vi "Read_WIP_All.vi"(7 "WIP In":i64[](array[numeric]), 8 "error in (no error)":errorcluster, 9 "WIP dIn":i64[](array[numeric]), 10 "Ref in":T1={"MS SQL Connection"=refnum, "UDL File"=path "", "Time"="", "DCODE"="", "WIP+1"=0, "MC No?"=0, "POKAYOKE?"=FALSE, "Expected Result"="", "Result [Status]"="", "Clock"=0.0, "RFID"="", "WIP Queue"=refnum, "TS Parameter"={"ProfitCenterCode"="", "LineCode"="", "WorkOrderNumber"="", "Model"="", "Model_with_Prefix"="", "VendorCode"="", "SetParameterDateCode"="", "PokaYoke"=0, "Target"=1, "Live_DateCode"="", "CustomerPartNumber"="", "Hand"="", "sBarcode"=FALSE, "FCA"=0, "Ent_Stamp"=timestamp(0 s since 1904-01-01), "STS_CD"=0.0}, "Data_Queue"=[], "RFID Serial No."=""} {"TS Parameter"."FCA" format="%01d"; "TS Parameter"."Target" min=1 max=100000; "TS Parameter"."PokaYoke" min=0 max=1}, 11 "Queue in":refnum<queue>) -> (0 "error out":errorcluster, 1 "WIP dOut":i64[](array[numeric]), 2 "Ref out":T1={"MS SQL Connection"=refnum, "UDL File"=path "", "Time"="", "DCODE"="", "WIP+1"=0, "MC No?"=0, "POKAYOKE?"=FALSE, "Expected Result"="", "Result [Status]"="", "Clock"=0.0, "RFID"="", "WIP Queue"=refnum, "TS Parameter"={"ProfitCenterCode"="", "LineCode"="", "WorkOrderNumber"="", "Model"="", "Model_with_Prefix"="", "VendorCode"="", "SetParameterDateCode"="", "PokaYoke"=0, "Target"=1, "Live_DateCode"="", "CustomerPartNumber"="", "Hand"="", "sBarcode"=FALSE, "FCA"=0, "Ent_Stamp"=timestamp(0 s since 1904-01-01), "STS_CD"=0.0}, "Data_Queue"=[], "RFID Serial No."=""} {"TS Parameter"."FCA" format="%01d"; "TS Parameter"."Target" min=1 max=100000; "TS Parameter"."PokaYoke" min=0 max=1}, 3 "Queue out":refnum<queue>, 4 "State Out":T4, 5 "WIP Out":i64[](array[numeric]))   [LabVIEW 2020]
uses:
  Controls/WIP_State.ctl
  Controls/TD SQL.ctl
  <vilib>/addons/database/Connection.llb/Conn ObjectReference.ctl
  Controls/TS_Parameter.ctl
  MS SQL/MS_Global.vi
  <vilib>/addons/database/NI_Database_API.lvlib
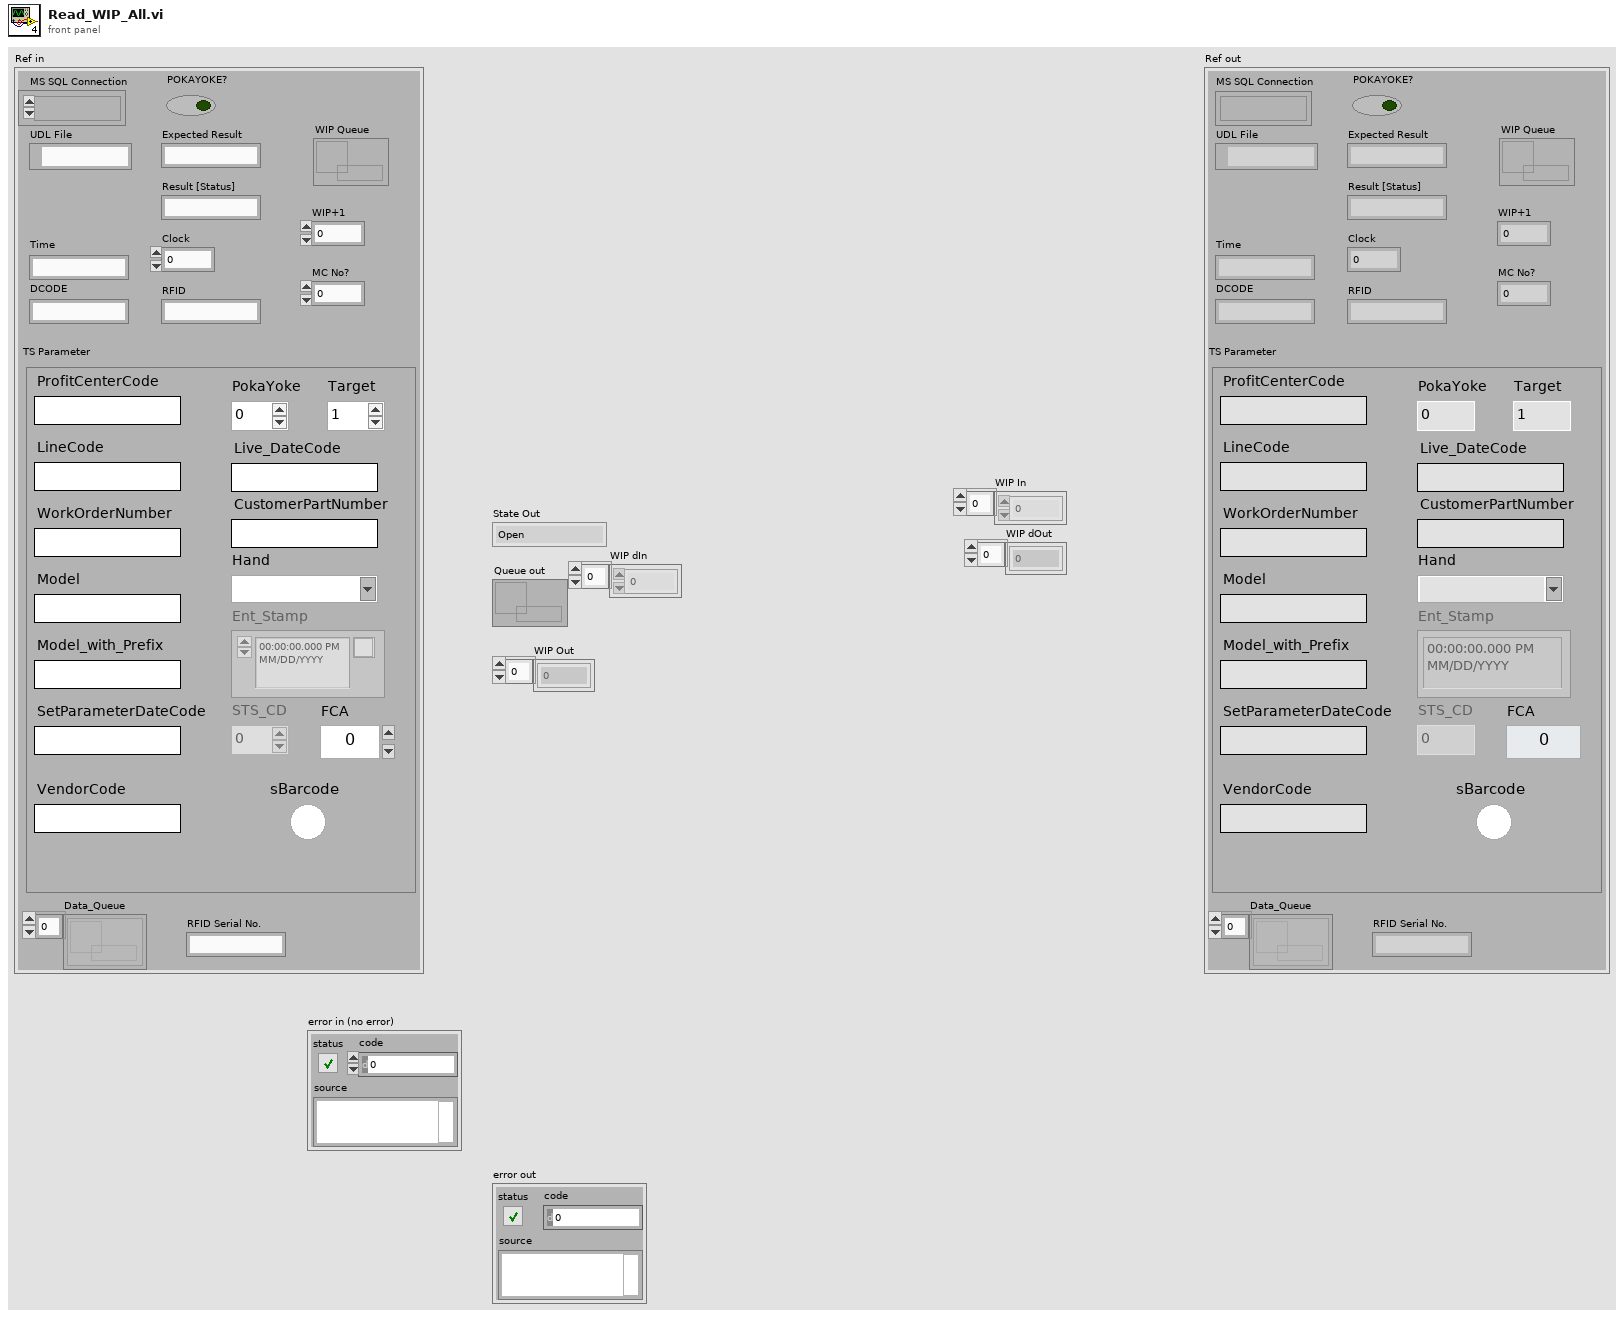
[diagram p1: front panel]
types:
  T1 = typedef "TD SQL.ctl" = cluster{"MS SQL Connection":T2, "UDL File":path, "Time":string, "DCODE":string, "WIP+1":i64, "MC No?":i32, "POKAYOKE?":bool, "Expected Result":string, "Result [Status]":string, "Clock":dbl, "RFID":string, "WIP Queue":refnum<queue>, "TS Parameter":T3, "Data_Queue":refnum<queue>[], "RFID Serial No.":string}
  T2 = typedef "NI_Database_API.lvlib/Conn ObjectReference.ctl" = refnum<k1>
  T3 = typedef "TS_Parameter.ctl" = cluster{"ProfitCenterCode":string, "LineCode":string, "WorkOrderNumber":string, "Model":string, "Model_with_Prefix":string, "VendorCode":string, "SetParameterDateCode":string, "PokaYoke":i32, "Target":i32, "Live_DateCode":string, "CustomerPartNumber":string, "Hand":string, "sBarcode":bool, "FCA":i32, "Ent_Stamp":timestamp, "STS_CD":dbl}
  T4 = typedef "WIP_State.ctl" = enum16{"Open", "Read", "Write", "Read WIP", "Flush", "Close"}
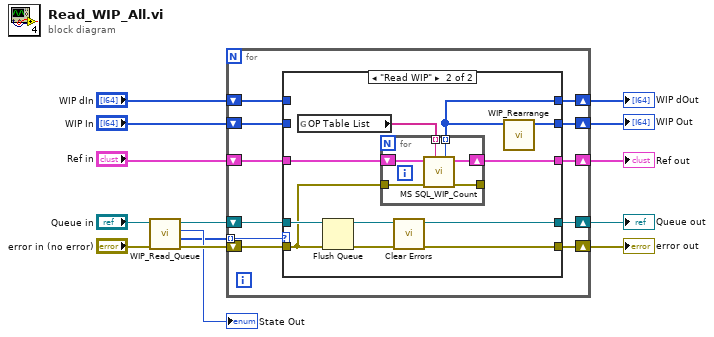
[diagram p0: block diagram]
diagram:
  n1 = call "WIP_Read_Queue.vi"("error in (no error)"="error in (no error)", "Queue In"="Queue in") -> ("error out"=w8:errorcluster, "State Out[]"=w3:T4[], "State Out"=→"State Out":T4, "Queue out"=w5:refnum<queue>)  [unwired: 6 in]
  n2 = for {
    shift-right: [w23] -> w11
    shift-left: "Ref in" -> [w22]
    shift-right: [w24] -> w12
    shift-left: w8 -> [w21]
    shift-right: [w18] -> w4
    shift-left: w5 -> [w19]
    tunnel: w3 -> [w17] mode=indexing
    shift-right: [w25] -> w13
    shift-left: "WIP In" -> [w20]
    shift-right: [w16] -> w1
    shift-left: "WIP dIn" -> [w15]
    n3 = case shown="\"Read WIP\"" w17 {
      tunnel: [w30 w32] -> w25
      tunnel: [w28 w35] -> w24
      tunnel: [w29 w40] -> w23
      tunnel: w22 -> [w29 w39]
      tunnel: w21 -> [w28 w33]
      tunnel: w20 -> [w30 _]
      tunnel: w19 -> [w27 w38]
      tunnel: [w27 w37] -> w18
      tunnel: [w26 w31] -> w16
      tunnel: w15 -> [w26 _]
      frame "Open", Default {
      }
      frame "Read WIP" {
        n4 = global read "MS_Global.vi" "OP Table List"() -> (w34:string[])
        n5 = Flush Queue(queue=w38, error in (no error)=w33) -> (queue out=w37:refnum<queue>, error out=w36:errorcluster)  [unwired: 1 out]
        n6 = for {
          tunnel: w33 -> [w45]
          shift-right: [w44] -> w40
          shift-left: w39 -> [w46]
          tunnel: [w43] -> _
          tunnel: w34 -> [w42] mode=indexing
          tunnel: [w41] -> w31 mode=indexing
          n7 = call "MS SQL_WIP_Count.vi"("Table"=w42, "error in (no error)"=w45, "Ref in"=w46) -> ("error out"=w43:errorcluster, "Ref Out"=w44:T1, "WIP"=w41:i64)  [unwired: 6 in]
        }
        n8 = call <vilib>:"Clear Errors.vi"("error in (no error)"=w36) -> ("error out"=w35:errorcluster)  [unwired: 5 in, 1 out]
        n9 = call "WIP_Rearrange.vi"("WIP in"=w31) -> ("WIP out"=w32:i64[])  [unwired: 10 in]
      }
    }
  }
  "Queue out" <- w4
  "WIP Out" <- w13
  "error out" <- w12
  "Ref out" <- w11
  "WIP dOut" <- w1
